vi "Write_Alicat_P_Control.vi"(6 "Current Set Point (NaN)":dbl=nan, 7 "Device ID (G)":string="G", 8 "error in (no error)":errorcluster, 9 "Device Range":dbl=500.0, 10 "Set Point":dbl, 11 "VISA Sesssion In":refnum<visa-resource-name>="ASRL6::INSTR") -> (0 "error out":errorcluster, 1 "read buffer":string, 2 "Serial Message":string, 3 "VISA Sesssion Out":refnum<visa-resource-name>="ASRL6::INSTR")   [LabVIEW 2019]
uses:
  <vilib>/Instr/_visa.llb/VISA Flush IO Buffer Mask.ctl
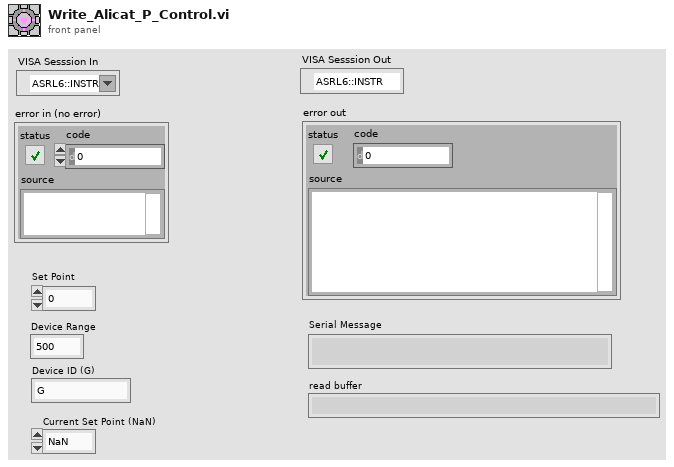
[diagram p1: front panel]
types:
  T1 = typedef "VISA Flush IO Buffer Mask.ctl" = u16
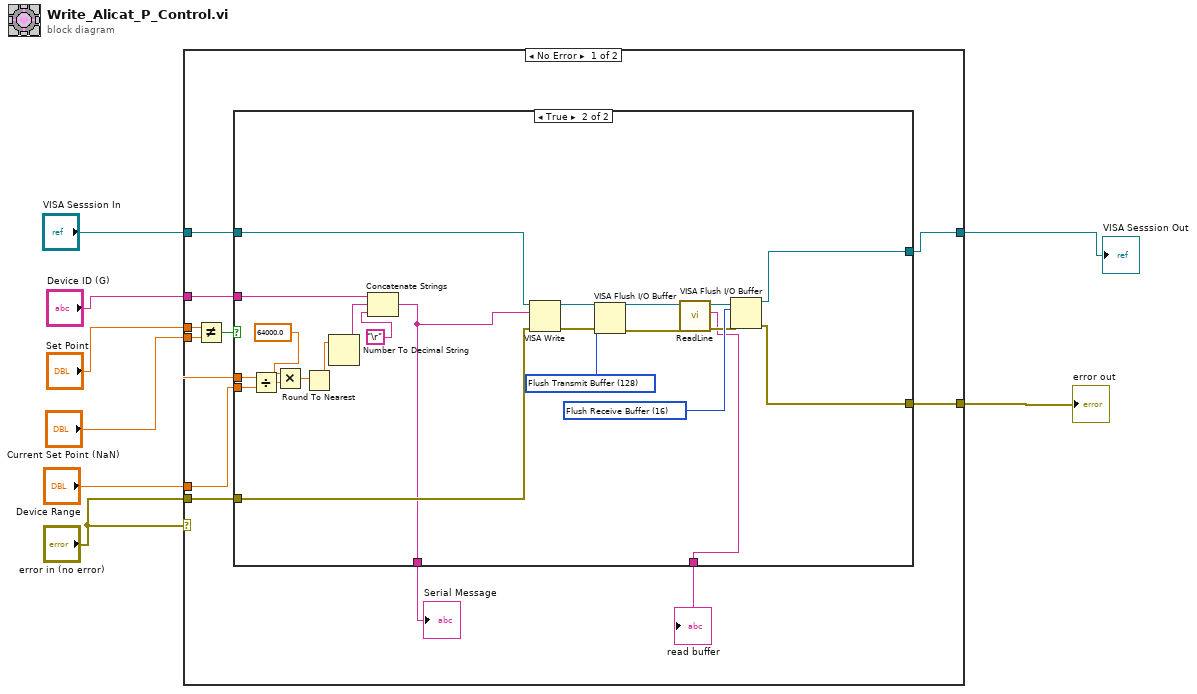
[diagram p0: block diagram]
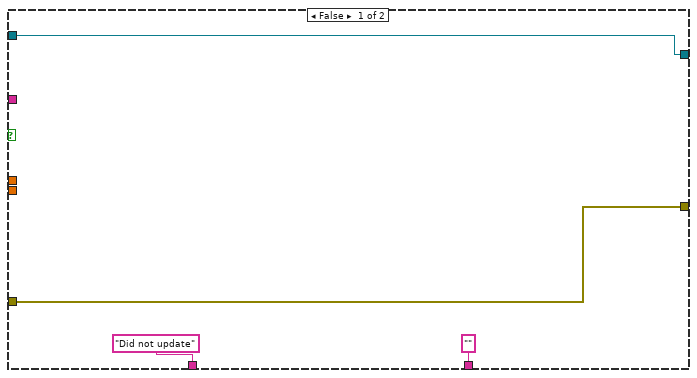
[diagram p2: hidden frame]
diagram:
  n1 = case shown="No Error" "error in (no error)" {
    tunnel: "Device ID (G)" -> [w19 _]
    tunnel: "error in (no error)" -> [w18 w48]
    tunnel: [w17 w48] -> w7
    tunnel: "Device Range" -> [w15 _]
    tunnel: "Set Point" -> [w14 _]
    tunnel: "Current Set Point (NaN)" -> [w11 _]
    tunnel: "VISA Sesssion In" -> [w10 w47]
    tunnel: [w9 w47] -> w1
    frame No Error {
      n2 = Not Equal?(x=w14, y=w11) -> (x != y?=w16:bool)
      n3 = case shown="True" w16 {
        tunnel: w14 -> [_ w41]
        tunnel: w15 -> [_ w40]
        tunnel: w19 -> [_ w39]
        tunnel: w10 -> [w20 w35]
        tunnel: w18 -> [w23 w34]
        tunnel: [w23 w33] -> w17
        tunnel: ["" ("read buffer") w26] -> w13
        tunnel: ["Did not update" w32] -> w12
        tunnel: [w20 w25] -> w9
        frame False {
        }
        frame True {
          w30 = T1 16 items=["Flush Receive Buffer"=16, "Write Transmit Buffer to Device"=32, "Flush Receive Buffer (No I/O)"=64, "Flush Transmit Buffer"=128] ("Mask")
          w31 = T1 128 items=["Flush Receive Buffer"=16, "Write Transmit Buffer to Device"=32, "Flush Receive Buffer (No I/O)"=64, "Flush Transmit Buffer"=128] ("Mask")
          n4 = Divide(x=w41, y=w40) -> (x/y=w43:dbl)
          n5 = Multiply(x=64000.0, y=w43) -> (x*y=w44:dbl)
          n6 = Round To Nearest(number=w44) -> (nearest integer value=w45:dbl)
          n7 = Number To Decimal String(number=w45) -> (decimal integer string=w46:string)  [unwired: 1 in]
          n8 = Concatenate Strings(w39, w46, "\r") -> (w32:string)
          n9 = VISA Write(VISA resource name=w35, write buffer=w32, error in (no error)=w34) -> (VISA resource name out=w38:refnum<visa-resource-name>, error out=w37:errorcluster)  [unwired: 1 out]
          n10 = VISA Flush I/O Buffer(VISA resource name=w38, mask (16)=w31, error in (no error)=w37) -> (VISA resource name out=w24:refnum<visa-resource-name>, error out=w29:errorcluster)
          n11 = call "ReadLine.vi"("error in (no error)"=w29, "VISA Sesssion In"=w24) -> ("error out"=w27:errorcluster, "Read Line"=w26:string, "VISA Sesssion Out"=w28:refnum<visa-resource-name>)  [unwired: 7 in]
          n12 = VISA Flush I/O Buffer(VISA resource name=w28, mask (16)=w30, error in (no error)=w27) -> (VISA resource name out=w25:refnum<visa-resource-name>, error out=w33:errorcluster)
        }
      }
      "read buffer" <- w13
      "Serial Message" <- w12
    }
    frame Error {
    }
  }
  "error out" <- w7
  "VISA Sesssion Out" <- w1
